vi "Auto Gas Switching 2.vi"() -> ()   [LabVIEW 2015]
uses:
  C:/Users/Narek/Desktop/h2scan/Auto Gas Switching/ULx_LV.dll
  ULx_LV.dll
  <vilib>/Utility/error.llb/DialogType.ctl
  <vilib>/ULx/Write.llb/ULx Write (Digital 1D Bool NChan 1Samp 1Line).vi
  <vilib>/ULx/Create Channel.llb/ULx Create Channel (DO-Digital Output).vi
  <vilib>/ULx/Timing.llb/ULx Timing (Sample Clock).vi
panel:
  out "Numeric 2":i32
  out "error out 2":errorcluster
  out "Time":i32
  out "error out":errorcluster
  out "task out":refnum<k24>
  out "Done":bool
  in  "Sel Gas":T1(radio)
  in  "Repeat":bool=TRUE
  out "Numeric":i32
  out "Step":i32
  in  "Table Control":string[][](table)=[["1"], ["2"], ["3"], ["4"], ["5"], ["6"], ["7"], ["8"], ["9"], ["10"], ["11"], ["12"], ["13"], ["14"], ["15"], ["16"], ["17"], ["18"], ["19"], ["20"], ["21"], ["22"], ["23"], ["24"], ["25"], ["26"], ["27"], ["28"]]
  out "Remaining":u32
  out "Gas":i32
  in  "stop":bool
  out "Set Gas":bool[](array[boolean])
  # "Auto Gas Switching"
  # "Version 2"
  # "The first time this program is run \nit could take 5-10 seconds to start"
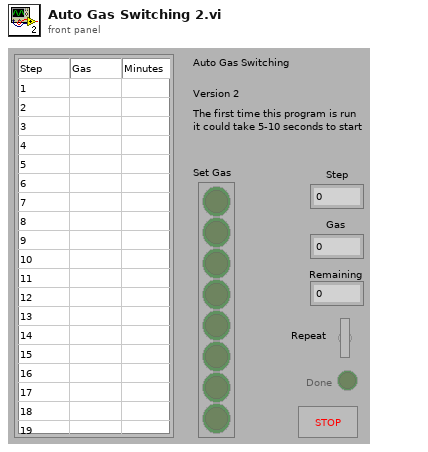
[diagram p1: front panel]
types:
  T1 = enum32{"Radio Selection 1", "Radio Selection 2", "Radio Selection 3", "Radio Selection 4", "Radio Selection 5"}
  T2 = typedef "DialogType.ctl" = u16
  T3 = enum8{"Enabled", "Disabled", "Disabled and Grayed Out"}
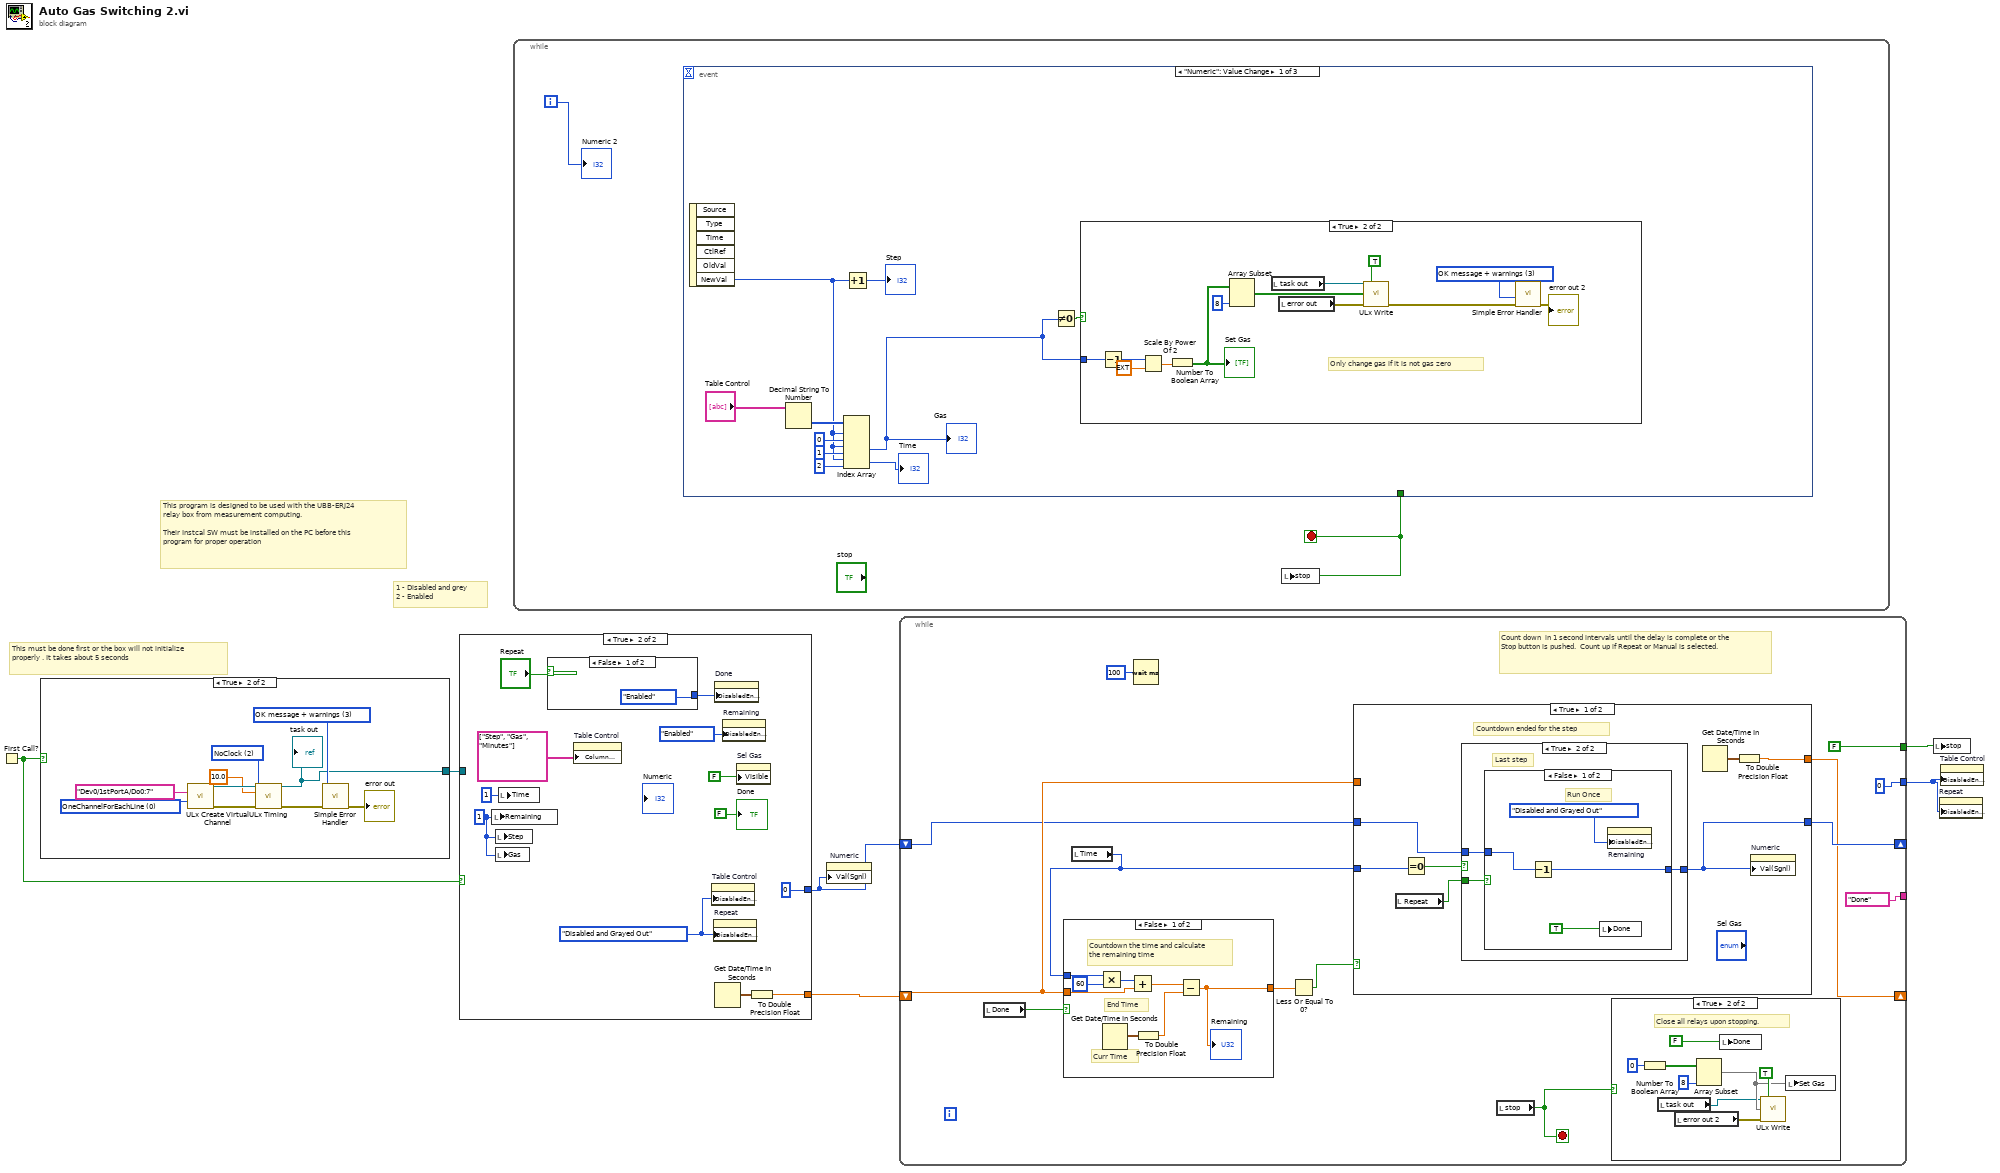
[diagram p0: block diagram]
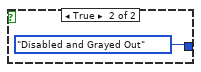
[diagram p4: hidden frame]
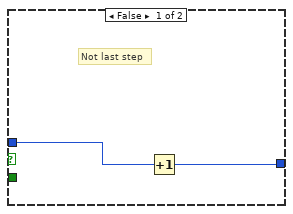
[diagram p7: hidden frame]
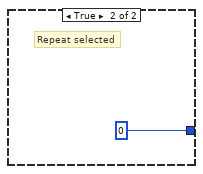
[diagram p8: hidden frame]
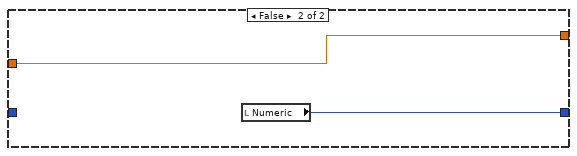
[diagram p9: hidden frame]
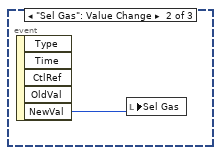
[diagram p11: hidden frame]
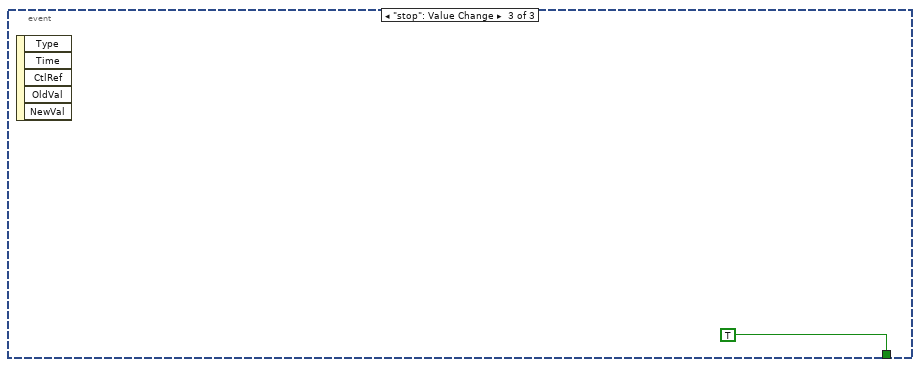
[diagram p12: hidden frame]
diagram:
  # "This program is designed to be used with the UBB-ERJ24 relay box from measurement computing.\n\nTheir Instcal SW must be installed on the PC before this program for proper operation"
  # "This must be done first or the box will not initialize properly . It takes about 5 seconds"
  # "1 - Disabled and grey\n2 - Enabled"
  n1 = First Call?() -> (First Call?: T/F=w3:bool)
  n2 = case shown="True" w3 {
    tunnel: [_ w7] -> w2
    frame False {
    }
    frame True {
      w8 = T2 3 items=["no dialog", "OK message", "continue or stop message", "OK message + warnings", "continue/stop + warnings"] ("type of dialog (OK msg:1)")
      w16 = 0 items=["OneChannelForEachLine", "OneChannelForAllLines"] ("line grouping")
      w14 = 2 items=["OnboardClock", "ExternalClock", "NoClock"] ("clock source")
      n3 = call-poly <vilib>:"ULx Create Virtual Channel.vi"("lines"="Dev0/1stPortA/Do0:7" ("string"), "line grouping"=w16) -> ("task out"=w12:refnum<k24>, "error out"=w13:errorcluster)  [unwired: 12 in]
      n4 = call-poly <vilib>:"ULx Timing.vi"("task in"=w12, "rate"=10.0, "clock source"=w14, "error in"=w13) -> ("task out"=w7:refnum<k24>, "error out"=w10:errorcluster)  [unwired: 10 in]
      "task out" <- w7
      n5 = call <vilib>:"Simple Error Handler.vi"("type of dialog (OK msg:1)"=w8, "error in (no error)"=w10) -> ("error out"=→"error out":errorcluster)  [unwired: 3 in, 4 out]
    }
  }
  n6 = case shown="True" w3 {
    tunnel: [_ w18] -> w5
    tunnel: [_ 0 ("Value (Signaling)")] -> w4
    tunnel: w2 -> [_ _]
    frame False {
    }
    frame True {
      w17 = T3."Disabled and Grayed Out" ("Disabled")
      w20 = u32 1 ("Remaining")
      n7 = local write "Remaining"(w20) -> ()
      n8 = local write "Step"(w20) -> ()
      n9 = local write "Gas"(w20) -> ()
      n10 = local write "Time"(1 ("Time")) -> ()
      n11 = case shown="False" "Repeat" {
        tunnel: [T3."Enabled" ("Disabled") T3."Disabled and Grayed Out" ("Disabled")] -> w22
        frame False {
        }
        frame True {
        }
      }
      n12 = property on="Table Control" class="Tbl (strict)"("Column Headers[]"=string[] ["Step", "Gas", "Minutes"] ("Row Header Strings[]")) -> ()  [unwired: 2 in, 2 out]
      n13 = property on="Table Control" class="Tbl (strict)"("DisabledEnum"=w17) -> ()  [unwired: 2 in, 2 out]
      n14 = property on="Repeat" class="Bool (strict)"("DisabledEnum"=w17) -> ()  [unwired: 2 in, 2 out]
      n15 = property on="Done" class="Bool (strict)"("DisabledEnum"=w22) -> ()  [unwired: 2 in, 2 out]
      n16 = Get Date/Time In Seconds() -> (seconds since 1Jan1904=w26:timestamp)
      n17 = property on="Remaining" class="DigNum (strict)"("DisabledEnum"=T3."Enabled" ("Disabled")) -> ()  [unwired: 2 in, 2 out]
      n18 = property on="Sel Gas" class="RadioBtnsControl (strict)"("Visible"=FALSE) -> ()  [unwired: 2 in, 2 out]
      n19 = To Double Precision Float(number=w26) -> (double precision float=w18:dbl)
      "Done" <- FALSE ("Done")
    }
  }
  n20 = while {
    i -> [w31]
    stop <- w32 stop-if-true
    n21 = event shown="[0] \"Numeric\": Value Change" {
      selector: _ -> [_ _ _]
      dyn-events: _ -> [_ _ _]
      timeout: _ -> [_ _ _]
      tunnel: [_ _ TRUE ("NewVal")] -> w32
      event "Numeric": Value Change {
        n22 = event-data() -> ("NewVal"=w34:i32)  [unwired: 1 in, 5 out]
        n23 = Decimal String To Number(string="Table Control") -> (number=w40:i32[][])  [unwired: 2 in, 1 out]
        n24 = Index Array(array=w40, index (row) #1=w34, index (col) #1=0 ("disabled index (col)"), index (row) #2=w34, index (col) #2=1 ("disabled index (col)"), index (row) #3=w34, index (col) #3=2 ("index (col)")) -> (element #2=w33:i32, element #3=→"Time":i32)  [unwired: 1 out]
        "Gas" <- w33
        n25 = Increment(x=w34) -> (x+1=→"Step":i32)
        n26 = Not Equal To 0?(x=w33) -> (x != 0?=w36:bool)
        n27 = case shown="True" w36 {
          tunnel: w33 -> [_ w43]
          frame False {
          }
          frame True {
            w49 = T2 3 items=["no dialog", "OK message", "continue or stop message", "OK message + warnings", "continue/stop + warnings"] ("type of dialog (OK msg:1)")
            # "Only change gas if it is not gas zero"
            n28 = Decrement(x=w43) -> (x-1=w52:i32)
            n29 = Scale By Power Of 2(n=w52, x=ext 1.0) -> (x*2^n=w44:ext)
            n30 = Number To Boolean Array(number=w44) -> (Boolean array=w50:bool[])
            "Set Gas" <- w50
            n31 = Array Subset(array=w50, length=8) -> (w55:bool[])  [unwired: 1 in]
            n32 = local read "task out"() -> (w48:refnum<k24>)
            n33 = local read "error out"() -> (w47:errorcluster)
            n34 = call-poly <vilib>:"ULx Write.vi"("task in"=w48, "auto start"=TRUE, "data"=w55, "error in"=w47) -> ("error out"=w46:errorcluster)  [unwired: 9 in, 2 out]
            n35 = call <vilib>:"Simple Error Handler.vi"("type of dialog (OK msg:1)"=w49, "error in (no error)"=w46) -> ("error out"=→"error out 2":errorcluster)  [unwired: 3 in, 4 out]
          }
        }
      }
      event "Sel Gas": Value Change {
        n36 = event-data() -> ("NewVal"=w56:T1)  [unwired: 1 in, 4 out]
        n37 = local write "Sel Gas"(w56) -> ()
      }
      event "stop": Value Change {
        n38 = event-data() -> ()  [unwired: 1 in, 5 out]
      }
    }
    n39 = local write "stop"(w32) -> ()
    "Numeric 2" <- w31
  }
  n40 = property on="Numeric" class="DigNum (strict)"("Val(Sgnl)"=w4) -> ()  [unwired: 2 in, 2 out]
  n41 = while {
    tunnel: [FALSE ("stop 2")] -> w6
    shift-right: [w69] -> _
    shift-left: w4 -> [w61]
    tunnel: [0 ("Numeric")] -> w1
    shift-right: [w67] -> _
    shift-left: w5 -> [w66]
    tunnel: ["Done" ("string")] -> _
    stop <- w62 stop-if-true
    # "Count down  in 1 second intervals until the delay is complete or the Stop button is pushed.  Count up if Repeat or Manual is selected."
    n42 = local read "Done"() -> (w64:bool)
    n43 = local read "Time"() -> (w63:i32)
    n44 = case shown="False" w64 {
      tunnel: w66 -> [w81 w87]
      tunnel: w63 -> [w80 _]
      tunnel: [w79 w87] -> w65
      frame False {
        # "Countdown the time and calculate the remaining time"
        # "Curr Time"
        # "End Time"
        n45 = Multiply(x=w80, y=60 ("x")) -> (x*y=w83:i32)
        n46 = Get Date/Time In Seconds() -> (seconds since 1Jan1904=w85:timestamp)
        n47 = Add(x=w83, y=w81) -> (x+y=w84:dbl)
        n48 = To Double Precision Float(number=w85) -> (double precision float=w82:dbl)
        n49 = Subtract(x=w84, y=w82) -> (x-y=w79:dbl)
        "Remaining" <- w79
      }
      frame True {
        # "Run once is complete, don't  change anything"
      }
    }
    n50 = Wait (ms)(milliseconds to wait=u32 100) -> ()  [unwired: 1 out]
    n51 = Less Or Equal To 0?(x=w65) -> (x <= 0?=w60:bool)
    n52 = case shown="True" w60 {
      tunnel: w61 -> [w90 _]
      tunnel: [w88 w106] -> w69
      tunnel: [w93 w105] -> w67
      tunnel: w66 -> [_ w105]
      tunnel: w63 -> [w92 _]
      frame True {
        # "Countdown ended for the step"
        n53 = local read "Repeat"() -> (w89:bool)
        n54 = Equal To 0?(x=w92) -> (x = 0?=w91:bool)
        n55 = case shown="True" w91 {
          tunnel: [w95 w99] -> w88
          tunnel: w90 -> [w96 w98]
          tunnel: w89 -> [_ w97]
          frame False {
            # "Not last step"
            n56 = Increment(x=w96) -> (x+1=w95:i32)
          }
          frame True {
            # "Last step"
            n57 = case shown="False" w97 {
              tunnel: [w100 0 ("t")] -> w99
              tunnel: w98 -> [w101 _]
              frame False {
                # "Run Once"
                n58 = Decrement(x=w101) -> (x-1=w100:i32)
                n59 = local write "Done"(TRUE ("Done")) -> ()
                n60 = property on="Remaining" class="DigNum (strict)"("DisabledEnum"=T3."Disabled and Grayed Out" ("Disabled")) -> ()  [unwired: 2 in, 2 out]
              }
              frame True {
                # "Repeat selected"
              }
            }
          }
        }
        n61 = Get Date/Time In Seconds() -> (seconds since 1Jan1904=w94:timestamp)
        n62 = To Double Precision Float(number=w94) -> (double precision float=w93:dbl)
        n63 = property on="Numeric" class="DigNum (strict)"("Val(Sgnl)"=w88) -> ()  [unwired: 2 in, 2 out]
      }
      frame False {
        n64 = local read "Numeric"() -> (w106:i32)
      }
    }
    n65 = local read "stop"() -> (w62:bool)
    n66 = case shown="True" w62 {
      frame False {
      }
      frame True {
        # "Close all relays upon stopping."
        n67 = Number To Boolean Array(number=0) -> (Boolean array=w76:bool[])
        n68 = local read "task out"() -> (w74:refnum<k24>)
        n69 = local read "error out 2"() -> (w73:errorcluster)
        n70 = Array Subset(array=w76, length=8) -> (w75:bool[])  [unwired: 1 in]
        n71 = local write "Done"(FALSE ("Done")) -> ()
        n72 = call-poly <vilib>:"ULx Write.vi"("task in"=w74, "auto start"=TRUE, "data"=w75, "error in"=w73) -> ()  [unwired: 9 in, 3 out]
        n73 = local write "Set Gas"(w75) -> ()
      }
    }
  }
  n74 = local write "stop"(w6) -> ()
  n75 = property on="Repeat" class="Bool (strict)"("DisabledEnum"=w1) -> ()  [unwired: 2 in, 2 out]
  n76 = property on="Table Control" class="Tbl (strict)"("DisabledEnum"=w1) -> ()  [unwired: 2 in, 2 out]
